vi "QueueRefs.vi"(7 "Set?":bool=TRUE, 10 "Queue Name":string, 11 "Queue Ref":refnum<queue>) -> (3 "Queue Ref":refnum<queue>)   [LabVIEW 2017, in "Message Queue.lvlib"]
uses:
  Message Queue.lvlib
  Message Cluster.ctl
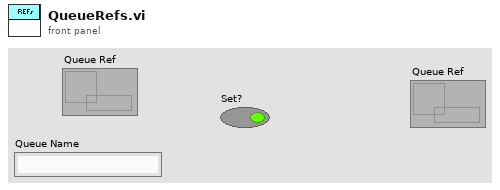
[diagram p1: front panel]
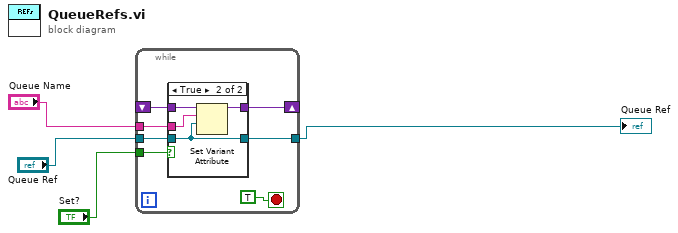
[diagram p0: block diagram]
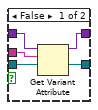
[diagram p2: hidden frame]
diagram:
  n1 = while {
    tunnel: "Queue Name" -> [w11]
    tunnel: "Set?" -> [w10]
    tunnel: "Queue Ref" -> [w8]
    shift-right: [w7] -> _
    shift-left: _ -> [w6]
    tunnel: [w5] -> w1
    stop <- TRUE stop-if-true
    n2 = case shown="True" w10 {
      tunnel: w11 -> [w14 w20]
      tunnel: w8 -> [w13 w17]
      tunnel: [w15 w19] -> w7
      tunnel: w6 -> [w16 w18]
      tunnel: [w12 w17] -> w5
      frame False {
        n3 = Get Variant Attribute(Variant=w16, name=w14, default value (empty Variant)=w13) -> (duplicate Variant=w15:variant, value=w12:refnum<queue>)  [unwired: 1 in, 2 out]
      }
      frame True {
        n4 = Set Variant Attribute(Variant=w18, name=w20, value=w17) -> (Variant out=w19:variant)  [unwired: 1 in, 2 out]
      }
    }
  }
  "Queue Ref" <- w1
